vi "Configure ARB Sequence Sweep Start Level.vi"(8 "error in":errorcluster, 10 "Value(HZ)":dbl min=0.0, 11 "VISA resource name":refnum<visa-resource-name>) -> (0 "error out":errorcluster, 3 "VISA resource name out":refnum<visa-resource-name>)   [LabVIEW 2024, in "IT-M3900C.lvlib"]
doc: "This command sets the starting frequency of the sweep signal in the sequence.\n<b>Value(HZ)</b>\nMIN-MAX"
uses:
  IT-M3900C.lvlib
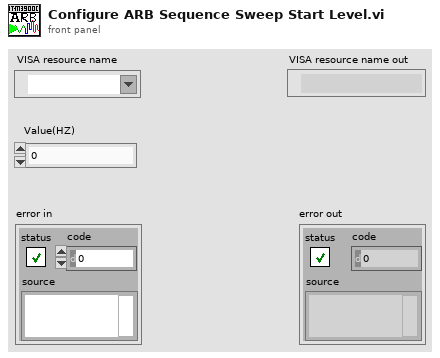
[diagram p1: front panel]
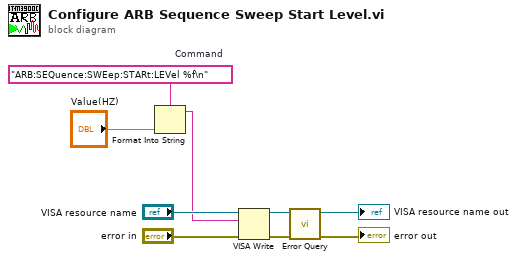
[diagram p0: block diagram]
diagram:
  w3 = "ARB:SEQuence:SWEep:STARt:LEVel %f\n"  # Command
  n1 = Format Into String(format string=w3, "Value(HZ)") -> (resulting string=w1:string)  [unwired: 2 in, 1 out]
  n2 = VISA Write(VISA resource name="VISA resource name", write buffer=w1, error in (no error)="error in") -> (VISA resource name out=w6:refnum<visa-resource-name>, error out=w7:errorcluster)  [unwired: 1 out]
  n3 = call "Error Query.vi"("error in"=w7, "VISA resource name"=w6) -> ("error out"=→"error out":errorcluster, "VISA resource name out"=→"VISA resource name out":refnum<visa-resource-name>)  [unwired: 6 in, 2 out]
